vi "SaveData.vi"(0 "object in":refnum<class "Application.lvclass">, 5 "error in (no error)":errorcluster) -> (14 "object out":refnum<class "Application.lvclass">, 19 "error out":errorcluster)   [LabVIEW 2019, in "Application.lvclass"]
uses:
  Application.lvclass
  MTec_class/MTec.lvclass
  InstrumentBase_class/AD2_SDK_class/InstrumentBase.lvclass
  Scheduler_class/Scheduler.lvclass
  AG34401Temperature_class/AG34401Temperature.lvclass
  MCCTemp_class/MCCTemp.lvclass
  TDMSLogger_class/TDMSLogger.lvclass
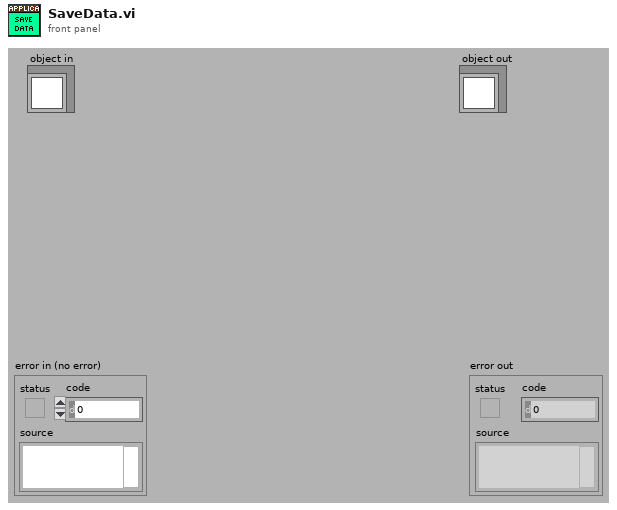
[diagram p1: front panel]
types:
  T1 = typedef "meTEC_ID 1200_Temperature is Stable.ctl" = i32
  T2 = typedef "meTEC_ID 104_Device Status.ctl" = i32
  T3 = cluster{"meTEC_CH2_Temperature Stability":T1, "meTEC_CH2_Act. Output Current [A]":dbl, "meTEC_CH2_Act. Output Voltage [V]":dbl, "meTEC_CH2_Object Temperature [°C]":dbl, "meTEC_CH2_Sink Temperature [°C]":dbl, "meTEC_CH1_Error Parameter":i32, "meTEC_CH1_Error Instance":i32, "meTEC_CH1_Error No.":i32, "meTEC_CH1_Device Status":T2, "meTEC_CH1_Temperature Stability":T1, "meTEC_CH1_Act. Output Current [A]":dbl, "meTEC_CH1_Act. Output Voltage [V]":dbl, "meTEC_CH1_Object Temperature [°C]":dbl, "meTEC_CH1_Sink Temperature [°C]":dbl}
  T4 = cluster{"Config.Ch1.Carrier.Frequency (Hz)":dbl, "Config.Ch2.Carrier.Frequency (Hz)":dbl, "Config.Ch1.Carrier.Amplitude (V)":dbl, "Config.Ch2.Carrier.Amplitude (V)":dbl}
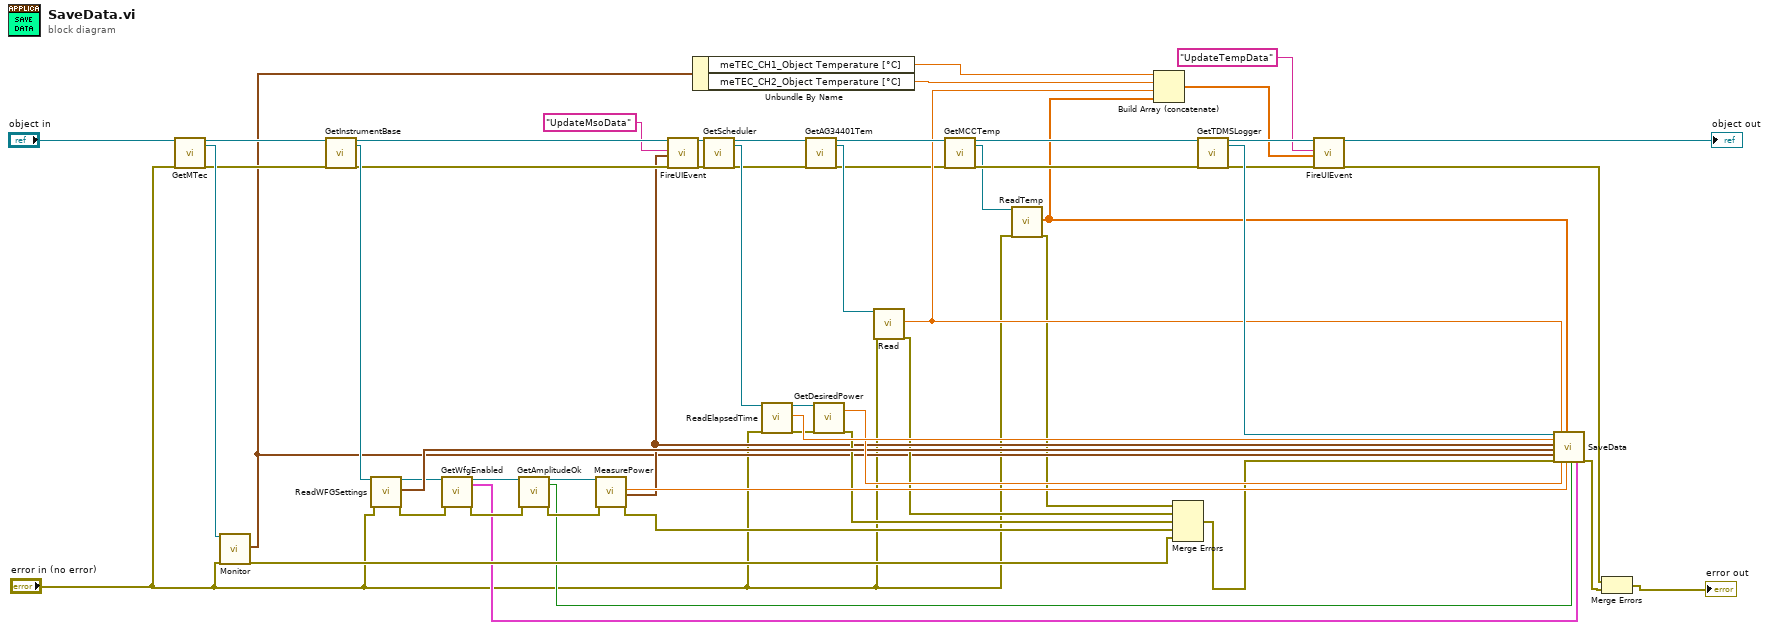
[diagram p0: block diagram]
diagram:
  n1 = call-dynamic "GetMTec.vi"("object in"="object in", "error in (no error)"="error in (no error)") -> ("object out"=w33:refnum<class "Application.lvclass">, "MTec"=w45:refnum<class "MTec.lvclass">, "error out"=w32:errorcluster)  [unwired: 15 in]
  n2 = call-dynamic "Monitor.vi"("object in"=w45, "error in (no error)"="error in (no error)") -> ("MtecData"=w12:T3, "error out"=w40:errorcluster)  [unwired: 15 in, 1 out]
  n3 = call-dynamic "GetInstrumentBase.vi"("object in"=w33, "error in (no error)"=w32) -> ("object out"=w39:refnum<class "Application.lvclass">, "InstrumentBase"=w47:refnum<class "InstrumentBase.lvclass">, "error out"=w37:errorcluster)  [unwired: 15 in]
  n4 = call-dynamic "ReadWFGSettings.vi"("object in"=w47, "error in (no error)"="error in (no error)") -> ("object out"=w30:refnum<class "InstrumentBase.lvclass">, "AmplitudeAndVoltage"=w48:T4, "error out"=w28:errorcluster)  [unwired: 15 in]
  n5 = call-dynamic "GetWfgEnabled.vi"("object in"=w30, "error in (no error)"=w28) -> ("object out"=w29:refnum<class "InstrumentBase.lvclass">, "WfgEnabled"=w23:cluster{"Ch1":bool, "Ch2":bool}, "error out"=w26:errorcluster)  [unwired: 15 in]
  n6 = call-dynamic "GetAmplitudeOk.vi"("object in"=w29, "error in (no error)"=w26) -> ("object out"=w27:refnum<class "InstrumentBase.lvclass">, "AmplitudeOk"=w24:bool, "error out"=w25:errorcluster)  [unwired: 15 in]
  n7 = call-dynamic "MeasurePower.vi"("object in"=w27, "error in (no error)"=w25) -> ("Measured Power"=w49:dbl, "Channels array"=w35:waveform(dbl)[], "error out"=w41:errorcluster)  [unwired: 14 in, 1 out]
  n8 = call-dynamic "FireUIEvent.vi"("object in"=w39, "Message"="UpdateMsoData", "Message Data"=w35, "error in (no error)"=w37) -> ("object out"=w38:refnum<class "Application.lvclass">, "error out"=w36:errorcluster)  [unwired: 14 in]
  n9 = Unbundle By Name(w12) -> ("meTEC_CH1_Object Temperature [°C]"=w11:dbl, "meTEC_CH2_Object Temperature [°C]"=w10:dbl)
  n10 = call-dynamic "GetScheduler.vi"("object in"=w38, "error in (no error)"=w36) -> ("object out"=w22:refnum<class "Application.lvclass">, "Scheduler"=w46:refnum<class "Scheduler.lvclass">, "error out"=w20:errorcluster)  [unwired: 15 in]
  n11 = call-dynamic "ReadElapsedTime.vi"("object in"=w46, "error in (no error)"="error in (no error)") -> ("object out"=w53:refnum<class "Scheduler.lvclass">, "Elapsed Time"=w52:dbl, "error out"=w50:errorcluster)  [unwired: 14 in, 1 out]
  n12 = call-dynamic "GetAG34401Tem.vi"("object in"=w22, "error in (no error)"=w20) -> ("object out"=w21:refnum<class "Application.lvclass">, "AG34401Tem"=w19:refnum<class "AG34401Temperature.lvclass">, "error out"=w6:errorcluster)  [unwired: 15 in]
  n13 = call-dynamic "GetDesiredPower.vi"("object in"=w53, "error in (no error)"=w50) -> ("DesiredPower"=w51:dbl, "error out"=w44:errorcluster)  [unwired: 15 in, 1 out]
  n14 = call-dynamic "Read.vi"("object in"=w19, "error in (no error)"="error in (no error)") -> ("GetTemp"=w9:dbl, "error out"=w18:errorcluster)  [unwired: 15 in, 1 out]
  n15 = call-dynamic "GetMCCTemp.vi"("object in"=w21, "error in (no error)"=w6) -> ("object out"=w7:refnum<class "Application.lvclass">, "MCCTemp"=w4:refnum<class "MCCTemp.lvclass">, "error out"=w5:errorcluster)  [unwired: 15 in]
  n16 = call-dynamic "ReadTemp.vi"("object in"=w4, "error in (no error)"="error in (no error)") -> ("data"=w1:dbl[], "error out"=w2:errorcluster)  [unwired: 15 in, 1 out]
  n17 = Build Array (concatenate)(w11, w10, w9, w1) -> (w8:dbl[])
  n18 = Merge Errors(w2, w18, w44, w41, w40) -> (w43:errorcluster)
  n19 = call-dynamic "GetTDMSLogger.vi"("object in"=w7, "error in (no error)"=w5) -> ("object out"=w15:refnum<class "Application.lvclass">, "TDMSLogger"=w54:refnum<class "TDMSLogger.lvclass">, "error out"=w17:errorcluster)  [unwired: 15 in]
  n20 = call-dynamic "FireUIEvent.vi"("object in"=w15, "Message"="UpdateTempData", "Message Data"=w8, "error in (no error)"=w17) -> ("object out"=→"object out":refnum<class "Application.lvclass">, "error out"=w16:errorcluster)  [unwired: 14 in]
  n21 = call-dynamic "SaveData.vi"("object in"=w54, "Elapsed Time"=w52, "ChannelsWFIn"=w35, "AmplitudeAndVoltageSettings"=w48, "MeTecData"=w12, "error in (no error)"=w43, "AGTemp"=w9, "SetPower"=w51, "MCCTempdata"=w1, "MeasuredPower"=w49, "AmplitudeOk"=w24, "WfgEnabled"=w23) -> ("error out"=w42:errorcluster)  [unwired: 6 in, 1 out]
  n22 = Merge Errors(w16, w42) -> (→"error out":errorcluster)
